vi "FanOnFromCloud.vi"() -> ()   [LabVIEW 2020]
uses:
  <vilib>/httpClient/LabVIEWHTTPClient.lvlib
panel:
  out "On/off":string
  out "FAN":u16(ring)
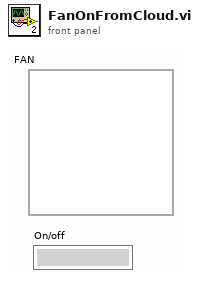
[diagram p1: front panel]
types:
  T1 = typedef "LabVIEWHTTPClient.lvlib/ClientHandle.ctl" = refnum<k1>
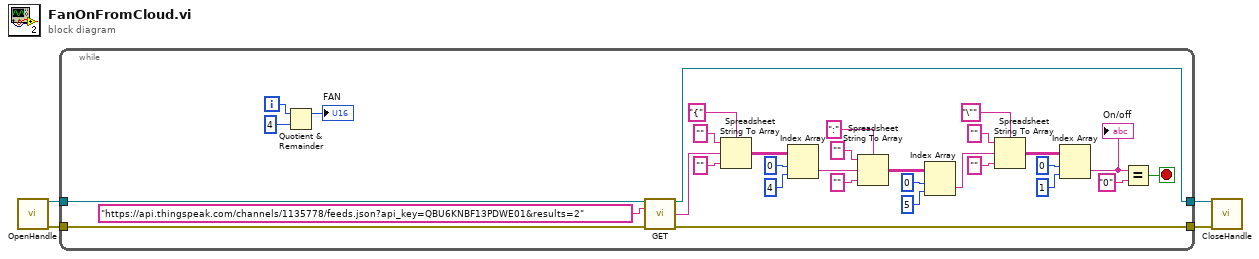
[diagram p0: block diagram]
diagram:
  n1 = call <vilib>:"OpenHandle.vi"() -> ("client handle out"=w3:T1, "error out"=w4:errorcluster)  [unwired: 14 in]
  n2 = while {
    tunnel: w4 -> [w36]
    tunnel: w3 -> [w33]
    tunnel: [w35] -> w2
    tunnel: [w29] -> w1
    i -> [w32]
    stop <- w5 stop-if-true
    n3 = Quotient & Remainder(x=w32, y=4) -> (x-y*floor(x/y)=→"FAN":i32)  [unwired: 1 out]
    n4 = call <vilib>:"GET.vi"("client handle"=w33, "url"="https://api.thingspeak.com/channels/1135778/feeds.json?api_key=QBU6KNBF13PDWE01&results=2", "error in (no error)"=w36) -> ("client handle out"=w29:T1, "body"=w28:string, "error out"=w35:errorcluster)  [unwired: 9 in, 1 out]
    n5 = Spreadsheet String To Array(delimiter (Tab)="{", format string="", spreadsheet string=w28, array type (2D Dbl)="") -> (array=w23:string[][])
    n6 = Index Array(array=w23, index (row)=0 ("index"), index (col)=4 ("disabled index (col)")) -> (element=w21:string)
    n7 = Spreadsheet String To Array(delimiter (Tab)=":", format string="", spreadsheet string=w21, array type (2D Dbl)="") -> (array=w17:string[][])
    n8 = Index Array(array=w17, index (row)=0, index (col)=5 ("disabled index (col)")) -> (element=w14:string)
    n9 = Spreadsheet String To Array(delimiter (Tab)="\"", format string="", spreadsheet string=w14, array type (2D Dbl)="") -> (array=w10:string[][])
    n10 = Index Array(array=w10, index (row)=0, index (col)=1 ("disabled index (col)")) -> (element=w7:string)
    "On/off" <- w7
    n11 = Equal?(x=w7, y="0") -> (x = y?=w5:bool)
  }
  n12 = call <vilib>:"CloseHandle.vi"("client handle"=w1, "error in (no error)"=w2) -> ()  [unwired: 13 in, 1 out]
